vi "Get nidaqmx_grpc_WriteDigitalLinesRequest.vi"(8 "error in (no error)":errorcluster, 11 "gRPCid":T1) -> (0 "error out":errorcluster, 2 "package_templatemessage":T2, 3 "gRPCid out":T1)   [LabVIEW 2021, in "NI DAQmx_server.lvlib"]
uses:
  NI DAQmx_server.lvlib
  nidaqmx_grpc_WriteDigitalLinesRequest.ctl
  nidevice_grpc_Session_session/nidevice_grpc_Session_session.lvclass
  nidaqmx_grpc_WriteDigitalLinesRequest_data_layout_enum/nidaqmx_grpc_WriteDigitalLinesRequest_data_layout_enum.lvclass
  nidevice_grpc_Session.ctl
  <vilib>/gRPC/LabVIEW gRPC Library/Shared/grpcId.ctl
  nidaqmx_grpc_WriteDigitalLinesRequest_Flat.ctl
  nidevice_grpc_Session_Flat.ctl
  nidaqmx_grpc_GroupBy.ctl
  nidevice_grpc_Session_session/nidevice_grpc_Session_session.lvclass/nidevice_grpc_Session_session.ctl
  nidaqmx_grpc_WriteDigitalLinesRequest_data_layout_enum/nidaqmx_grpc_WriteDigitalLinesRequest_data_layout_enum.lvclass/nidaqmx_grpc_WriteDigitalLinesRequest_data_layout_enum.ctl
  2ed25e12-861d-4677-8ead-ace2906b2041.vi
  <vilib>/gRPC/LabVIEW gRPC Library/Shared/TranslateGrpcError.vi
  FlatToRichnidevice_grpc_Session.vi
  nidaqmx_grpc_WriteDigitalLinesRequest_data_layout_enum/Setdata_layout.vi
  nidaqmx_grpc_WriteDigitalLinesRequest_data_layout_enum/Setdata_layout_raw.vi
  nidevice_grpc_Session_session/Setname.vi
  nidevice_grpc_Session_session/Setid.vi
  <vilib>/gRPC/LabVIEW gRPC Library/Server API/Server/Get Server DLL Path.vi
  <vilib>/Utility/error.llb/Error Cluster From Error Code.vi
  nidaqmx_grpc_WriteDigitalLinesRequest_data_layout_enum/GetFieldFromProtobufIndexnidaqmx_grpc_WriteDigitalLinesRequest_data_layout_enum.vi
  nidevice_grpc_Session_session/GetFieldFromProtobufIndexnidevice_grpc_Session_session.vi
  <vilib>/gRPC/LabVIEW gRPC Library/grpc-lvsupport-release.lvlib
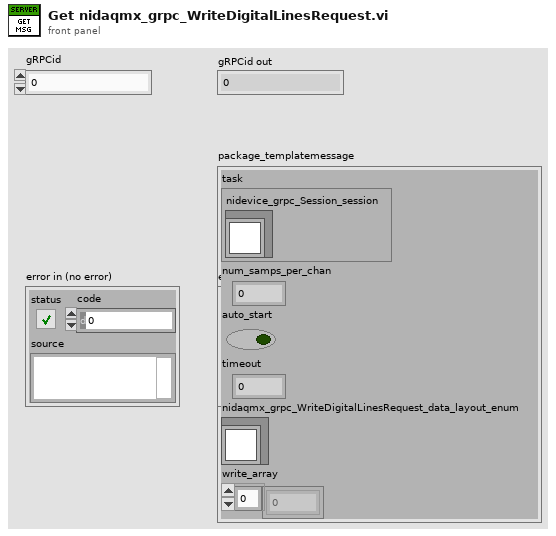
[diagram p1: front panel]
types:
  T1 = typedef "grpc-lvsupport-release.lvlib/grpcId.ctl" = u64
  T2 = typedef "NI DAQmx_server.lvlib/nidaqmx_grpc_WriteDigitalLinesRequest.ctl" = cluster{"task":T3, "num_samps_per_chan":i32, "auto_start":bool, "timeout":dbl, "nidaqmx_grpc_WriteDigitalLinesRequest_data_layout_enum":refnum<class "nidaqmx_grpc_WriteDigitalLinesRequest_data_layout_enum.lvclass">, "write_array":u8[]}
  T3 = typedef "NI DAQmx_server.lvlib/nidevice_grpc_Session.ctl" = cluster{"nidevice_grpc_Session_session":refnum<class "nidevice_grpc_Session_session.lvclass">}
  T4 = typedef "NI DAQmx_server.lvlib/nidaqmx_grpc_WriteDigitalLinesRequest_Flat.ctl" = cluster{"task":T5, "num_samps_per_chan":i32, "auto_start":bool, "timeout":dbl, "nidaqmx_grpc_WriteDigitalLinesRequest_data_layout_enum_selected_index":i32, "data_layout":T6, "data_layout_raw":i32, "write_array":u8[]}
  T5 = typedef "NI DAQmx_server.lvlib/nidevice_grpc_Session_Flat.ctl" = cluster{"nidevice_grpc_Session_session_selected_index":i32, "name":string, "id":u32}
  T6 = typedef "NI DAQmx_server.lvlib/nidaqmx_grpc_GroupBy.ctl" = enum32{"GROUP_BY_GROUP_BY_CHANNEL", "GROUP_BY_GROUP_BY_SCAN_NUMBER"}
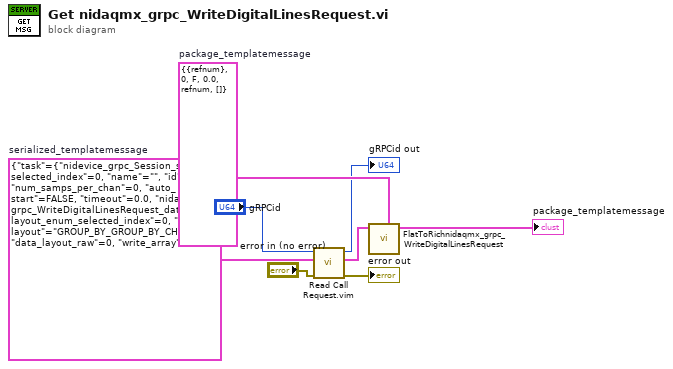
[diagram p0: block diagram]
diagram:
  w6 = T4 {"task"={"nidevice_grpc_Session_session_selected_index"=0, "name"="", "id"=0}, "num_samps_per_chan"=0, "auto_start"=FALSE, "timeout"=0.0, "nidaqmx_grpc_WriteDigitalLinesRequest_data_layout_enum_selected_index"=0, "data_layout"=enum."GROUP_BY_GROUP_BY_CHANNEL", "data_layout_raw"=0, "write_array"=[]}  # serialized_templatemessage
  w5 = T2 {"task"={"nidevice_grpc_Session_session"=refnum}, "num_samps_per_chan"=0, "auto_start"=FALSE, "timeout"=0.0, "nidaqmx_grpc_WriteDigitalLinesRequest_data_layout_enum"=refnum, "write_array"=[]}  # package_templatemessage
  n1 = call "Read Call Request.vim"("error in"="error in (no error)", "Request Type"=w6, "gRPCid in"="gRPCid") -> ("error out"=→"error out":errorcluster, "Request Data"=w4:T4, "gRPCid out"=→"gRPCid out":T1)  [unwired: 6 in]
  n2 = call "FlatToRichnidaqmx_grpc_WriteDigitalLinesRequest.vi"("OutputClusterType"=w5, "InputCluster"=w4) -> ("OutputCluster"=→"package_templatemessage":T2)  [unwired: 9 in]
